vi "Get Resource ID.vi"(4 "Resource in":refnum<class "Resource.lvclass">) -> (7 "Resource ID":string)   [LabVIEW 2024, in "CTI.lvlib" / "Resource.lvclass"]
uses:
  Resource.lvclass
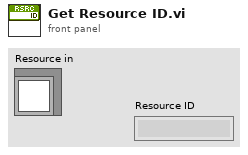
[diagram p1: front panel]
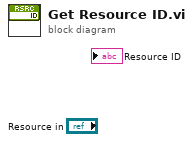
[diagram p0: block diagram]
diagram:
